vi "TSM SSC Digital Read Sequencer Register.vi"(0 "Digital TSM in":T1, 5 "Sequencer Register":string(combo)="reg0", 11 "error in":errorcluster) -> (4 "Digital TSM out":T1, 6 "Per-Instrument Register Values":i32[](array[numeric]), 15 "error out":errorcluster)   [LabVIEW 2020]
doc: "Reads the value of a pattern sequencer register on the device(s) connected to the specified pin(s) and pin group(s). Use pattern sequencer registers to pass numeric values between the pattern sequencer and a runtime test program."
uses:
  TSM/TSM SSC Digital.ctl
  <vilib>/NI_TestStand_SemiconductorModule/NI_TestStand_Semiconductor_Module.lvlibp/PinMap/Digital Pattern/PinQueryContext/DigitalPatternPinQueryContext.lvclass
  SSC Digital/SSC Digital.ctl
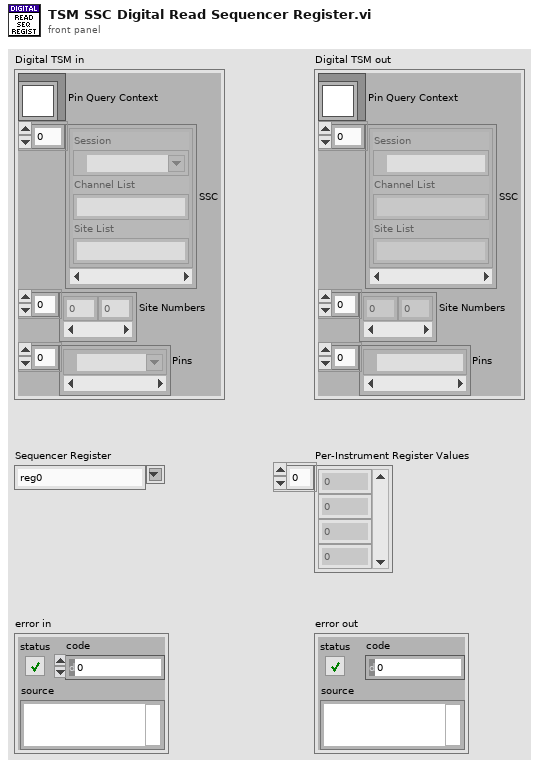
[diagram p1: front panel]
types:
  T1 = typedef "TSM SSC Digital.ctl" = cluster{"Pin Query Context":refnum<class "DigitalPatternPinQueryContext.lvclass">, "SSC":T2[], "Site Numbers":i32[], "Pins":tag[]}
  T2 = typedef "SSC Digital.ctl" = cluster{"Session":refnum<k15>, "Channel List":string, "Site List":string}
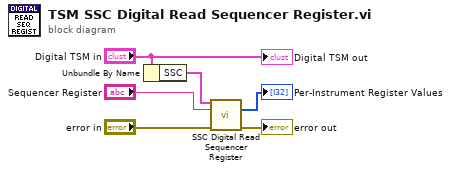
[diagram p0: block diagram]
diagram:
  n1 = Unbundle By Name("Digital TSM in") -> ("SSC"=w5:T2[])
  n2 = call "SSC Digital Read Sequencer Register.vi"("Digital SSC in"=w5, "Sequencer Register"="Sequencer Register", "error in"="error in") -> ("Per-Instrument Register Values"=→"Per-Instrument Register Values":i32[], "error out"=→"error out":errorcluster)  [unwired: 10 in, 1 out]
  "Digital TSM out" <- "Digital TSM in"
